vi "initialize_currents.vi"(8 "error in 2":errorcluster, 10 "Device Handle Out":u32, 11 "REACTORS":T1) -> (0 "ERROR OUT":errorcluster, 2 "Device Handle Out 2":u32, 3 "REACTORS 2":T1)   [LabVIEW 2013]
uses:
  type_defs/reactor.ctl
  type_defs/reactors.ctl
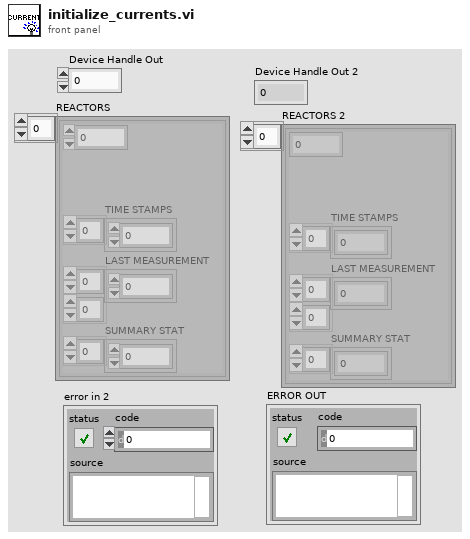
[diagram p1: front panel]
types:
  T1 = typedef "reactors.ctl" = cluster{i32, "TIME STAMPS":dbl[], "LAST MEASUREMENT":T2[][], "SUMMARY STAT":dbl[]}[]
  T2 = typedef "reactor.ctl" = dbl
  T3 = enum16{"Set Mode", "Set Normal Current ", "Set Strobe Parameters", "Set Normal Parameters", "Set Strobe Profile "}
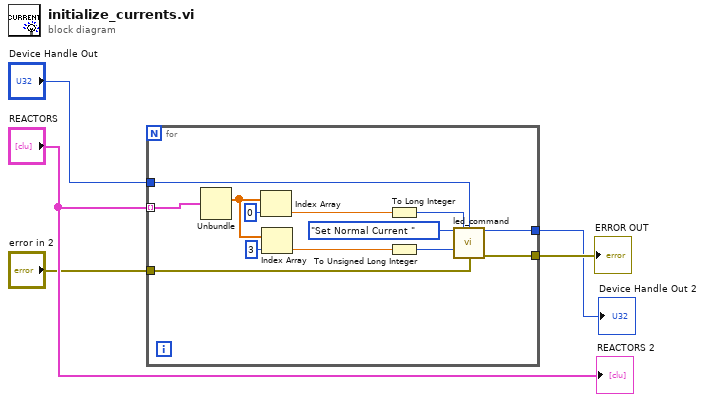
[diagram p0: block diagram]
diagram:
  n1 = for {
    tunnel: "REACTORS" -> [w15] mode=indexing
    tunnel: "Device Handle Out" -> [w13]
    tunnel: "error in 2" -> [w8]
    tunnel: [w7] -> w2
    tunnel: [w6] -> w1
    n2 = Unbundle(w15) -> ("TIME STAMPS"=w16:dbl[])  [unwired: 3 out]
    n3 = Index Array(array=w16, index=0) -> (element=w14:dbl)
    n4 = Index Array(array=w16, index=3) -> (element=w11:dbl)
    n5 = To Long Integer(number=w14) -> (32bit integer=w10:i32)
    n6 = To Unsigned Long Integer(number=w11) -> (unsigned 32bit integer=w9:u32)
    n7 = call "led_command.vi"("COMMAND"=T3."Set Normal Current ", "Channel"=w10, "Device Handle"=w13, "Iset"=w9, "ERROR"=w8) -> ("Device Handle Out"=w6:u32, "ERROR OUT"=w7:errorcluster)  [unwired: 7 in, 2 out]
  }
  "ERROR OUT" <- w2
  "Device Handle Out 2" <- w1
  "REACTORS 2" <- "REACTORS"
